vi "Enable Control.vi"(7 "Select Channel":i32=1 min=1 max=4 step=1, 8 "error in (no error)":errorcluster, 10 "Enable Control":bool, 11 "Lakeshore 336 in":refnum<class "Lakeshore 336.lvclass">) -> (0 "error out":errorcluster, 3 "Lakeshore 336 out":refnum<class "Lakeshore 336.lvclass">)   [LabVIEW 2022 SP3, in "Lakeshore 336.lvclass"]
uses:
  Lakeshore 336.lvclass
  Lakeshore 336.lvclass/Lakeshore 336.ctl
  Temp Control.lvclass
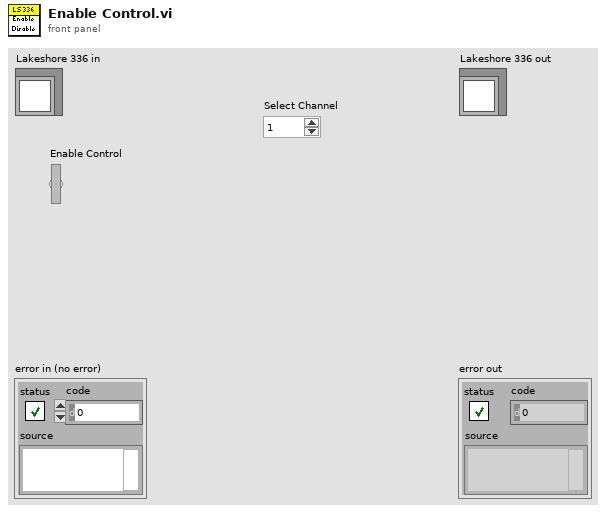
[diagram p1: front panel]
types:
  T1 = typedef "Lakeshore 336.lvclass/Lakeshore 336 Channel Settings cluster.ctl" = cluster{"Input (0:None)":u16, "Power Up Enable (F: Off)":bool, "Mode (0:Off)":u16, "Max Current (0:User Specified)":u16, "Heater Out Display (1:Current)":u16, "Max User Current (2.000)":dbl, "Heater Resistance (1:25 Ohms)":u16, "PID":T2, "Name":string}
  T2 = typedef "Lakeshore 336.lvclass/Lakeshore 336 PID cluster.ctl" = cluster{"P":dbl, "I":dbl, "D":dbl}
  T3 = typedef "Lakeshore 336.lvclass/Lakeshore 336 Settings cluster.ctl" = cluster{"Lake Shore 336 Address":refnum<visa-resource-name>, "Output Ch":T1[], "Input Ch":T4[], "Prefix":string, "Setpoints":dbl[], "Control Enable":bool[]}
  T4 = typedef "Lakeshore 336.lvclass/Lakeshore 336 Input Ch config cluster.ctl" = cluster{"Name":string}
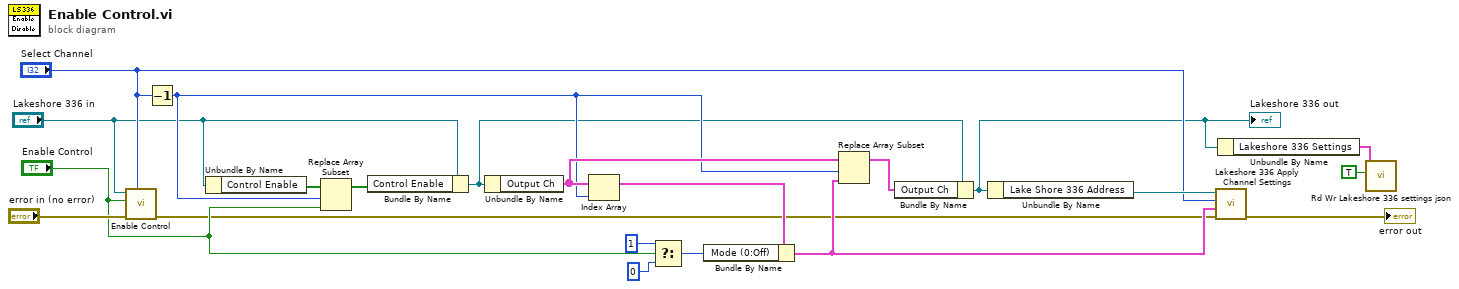
[diagram p0: block diagram]
diagram:
  n1 = call-parent "Enable Control.vi"("Select Channel"="Select Channel", "error in (no error)"="error in (no error)", "Enable Control"="Enable Control", "Temp Control in"="Lakeshore 336 in") -> ("error out"=w8:errorcluster)  [unwired: 6 in, 1 out]
  n2 = Decrement(x="Select Channel") -> (x-1=w6:i32)
  n3 = Unbundle By Name("Lakeshore 336 in") -> ("Control Enable"=w20:bool[])
  n4 = Replace Array Subset(array=w20, new element="Enable Control", index=w6) -> (w19:bool[])
  n5 = Bundle By Name(cluster="Lakeshore 336 in", "Control Enable"=w19) -> (w2:refnum<class "Lakeshore 336.lvclass">)
  n6 = Unbundle By Name(w2) -> ("Output Ch"=w13:T1[])
  n7 = Index Array(array=w13, index=w6) -> (element=w15:T1)
  n8 = Select(t=u16 1, s="Enable Control", f=u16 0 ("Mode (0:Off)")) -> (s? t:f=w17:u16)
  n9 = Bundle By Name(cluster=w15, "Mode (0:Off)"=w17) -> (w10:T1)
  n10 = Replace Array Subset(array=w13, new element=w10, index=w6) -> (w12:T1[])
  n11 = Bundle By Name(cluster=w2, "Output Ch"=w12) -> (w1:refnum<class "Lakeshore 336.lvclass">)
  "Lakeshore 336 out" <- w1
  n12 = Unbundle By Name(w1) -> ("Lake Shore 336 Address"=w11:refnum<visa-resource-name>)
  n13 = call "Lakeshore 336 Apply Channel Settings.vi"("error in (no error)"=w8, "Manual Settings"=w10, "Channel (1)"="Select Channel", "Addr"=w11) -> ("error out"=→"error out":errorcluster)  [unwired: 5 in, 2 out]
  n14 = Unbundle By Name(w1) -> ("Lakeshore 336 Settings"=w5:T3)
  n15 = call "Rd Wr Lakeshore 336 settings json.vi"("Write? (F:Read)"=TRUE, "Lakeshore 336 Settings"=w5) -> ()  [unwired: 8 in, 2 out]
